vi "Send Stop.vi"(8 "error in (no error)":errorcluster, 11 "UI in":refnum<class "UI.lvclass">) -> (0 "error out":errorcluster)   [LabVIEW 2020, in "AR Example.lvlib" / "UI.lvclass"]
uses:
  UI.lvclass
  <vilib>/event_ctls.llb/usereventprio.ctl
  Stop Event.ctl
  UI.lvclass/UI.ctl
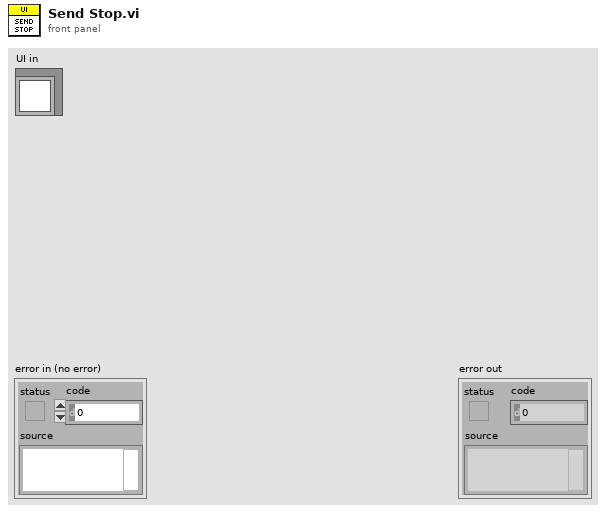
[diagram p1: front panel]
types:
  T1 = typedef "AR Example.lvlib/UI.lvclass/Stop Event.ctl" = cluster{"Data":bool}
  T2 = typedef "usereventprio.ctl" = enum32{"high priority", "normal priority"}
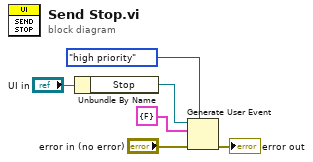
[diagram p0: block diagram]
diagram:
  n1 = Unbundle By Name("UI in") -> ("Stop"=w5:refnum<user-event>)
  n2 = Generate User Event(priority (normal)=usereventprio."high priority", user event=w5, event data cluster=T1 {"Data"=FALSE} ("event data"), error in="error in (no error)") -> (error out=→"error out":errorcluster)  [unwired: 1 out]
